vi "mongo_cursor_next.vi"(11 "cursor ptr":u32) -> (2 "return type":i32, 3 "cursor ptr out":u32)   [LabVIEW 2013]
uses:
  mongo-c-driver/libmongoc.so
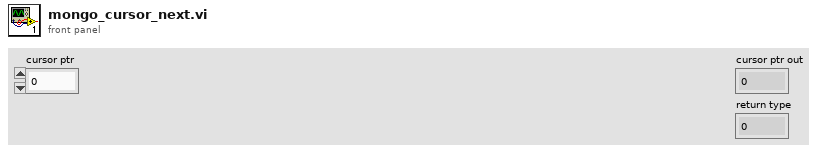
[diagram p1: front panel]
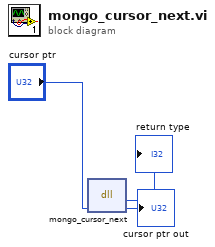
[diagram p0: block diagram]
diagram:
  n1 = dll-call lib="home/scot/dev/git/mongo-c-driver/libmongoc.so" fn="mongo_cursor_next"("cursor ptr"="cursor ptr") -> ("return type"=→"return type":i32, "cursor ptr"=→"cursor ptr out":u32)  [unwired: 3 in, 2 out]
